vi "CrudeDataReader.vi"() -> ()   [LabVIEW 2016]
panel:
  in  "Filename":path=path "D:/Sonify Labview/Data/PorkSkin_40C_5Min.lvm"
  out "Signals":dynamicdata(graph)
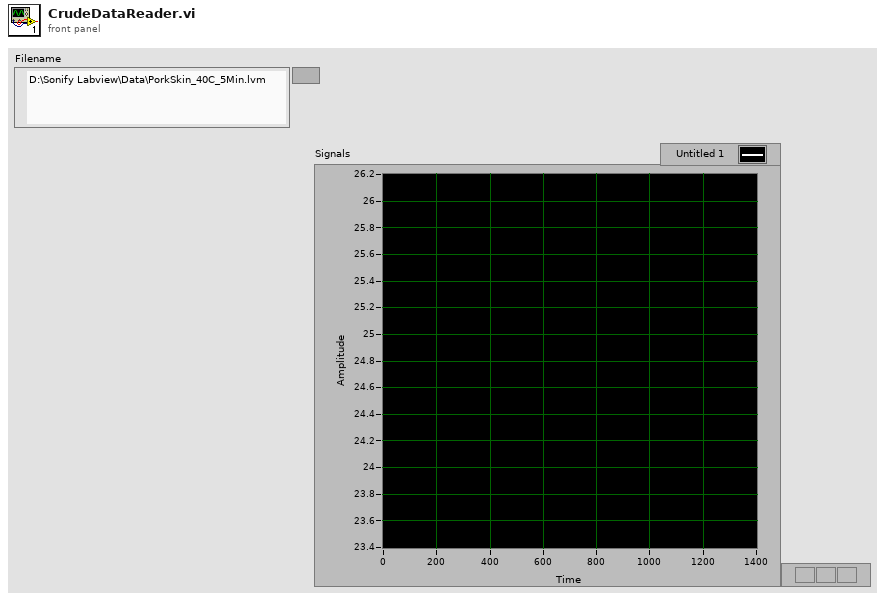
[diagram p1: front panel]
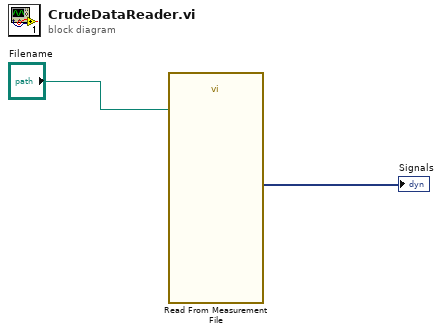
[diagram p0: block diagram]
diagram:
  n1 = call "Read From Measurement File"("Filename"="Filename") -> ("Signals"=→"Signals":dynamicdata)  [unwired: 5 in, 5 out]
